vi "gVar_ECa4.vi"() -> ()   [LabVIEW 2020]
panel:
  out "ECa4":dbl
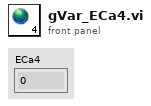
[diagram p1: front panel]
diagram:
